vi "ERR Error Handler.vi"(0 "Error Status":bool, 5 "Error Code":i32, 7 "Cause Of Error":string, 9 "Error Source In":string="SubVI", 11 "Error In (no error)":errorcluster, 12 "Previous Error In (no Error)":errorcluster={"status"=FALSE, "code"=0, "source"="Empty"}) -> (15 "Error Out":errorcluster)   [LabVIEW 2012]
doc: "This VI has two modes: Error Handler Mode, and User Error Mode.\nWhen the error flag is FALSE then the vi functions as an error has not ocurred then the error cluster is passed through. If an error has ocurred then it will handle the error. If a previous error has not ocurred and the Error Flag is TRUE then the VI will assert the error and pass it through.\n\nUpon asserting a user error the vi checks to see if the New Error Code corresponds to one in the initialized error code array if it does not find it then it will use error code 9999 and state the \"Error Not In Error File\" message within the source text. This may be because of an incorrect error code, an error code not entered in the ErrorDescription.ini file or an unitialized error operation.\n\nThe error source will contain the date, time, error description, cause of error (if entered), and the call chain of the error occurrence.\n\nIf an error is flagged that is not present in the error description file (e.g., it is a labview error) then an automatic dialog box is opened. If a user error is found then a dialog box will be opened only if the error level is not '0'. If the error level is greater than 1 then the error handling is bypassed (i.e., the error is not recovered and is passed though).\n\nThe error will be logged always or the first time it is handled in pass through mode (level=0).\n\nIf the erro level is '2' then a 3 button dialog will be called in order for the user to select: Recover, Pass Through, or Stop. The VI will log the users selection as well as any additional comments in the recovery line of the error log. It will then take the appropriate action depending on the dialog choice.\n\nThis vi was created by David Gianetto, contact me with any problems, questions, etc."
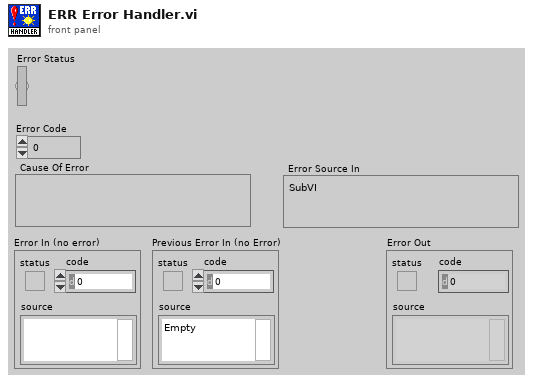
[diagram p1: front panel]
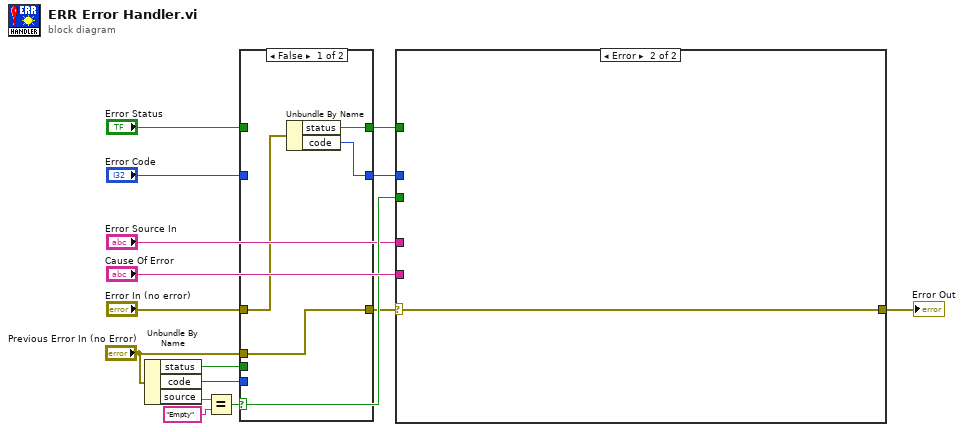
[diagram p0: block diagram]
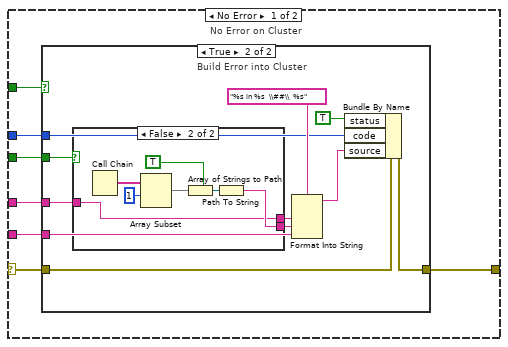
[diagram p3: hidden frame]
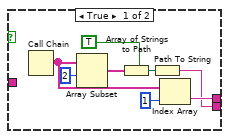
[diagram p5: hidden frame]
diagram:
  n1 = Unbundle By Name("Previous Error In (no Error)") -> ("status"=w7:bool, "code"=w6:i32, "source"=w13:string)
  n2 = Equal?(x=w13, y="Empty") -> (x = y?=w5:bool)
  n3 = case shown="False" w5 {
    tunnel: [w16 w22] -> w3
    tunnel: "Error Status" -> [_ w22]
    tunnel: [w17 w21] -> w2
    tunnel: "Error Code" -> [_ w21]
    tunnel: [w19 w20] -> w1
    tunnel: "Error In (no error)" -> [w18 w20]
    tunnel: w7 -> [_ _]
    tunnel: w6 -> [_ _]
    tunnel: "Previous Error In (no Error)" -> [w19 _]
    frame False {
      n4 = Unbundle By Name(w18) -> ("status"=w16:bool, "code"=w17:i32)
    }
    frame True {
    }
  }
  n5 = case shown="Error" w1 {
    selector: w1 -> [w23 w57]
    tunnel: [w27 w57] -> w15
    tunnel: w3 -> [w26 _]
    tunnel: w2 -> [w29 _]
    tunnel: "Cause Of Error" -> [w28 _]
    tunnel: w5 -> [w25 _]
    tunnel: "Error Source In" -> [w24 _]
    frame No Error {
      # "No Error on Cluster"
      n6 = case shown="True" w26 {
        tunnel: w29 -> [_ w34]
        tunnel: w28 -> [_ w33]
        tunnel: [errorcluster {"status"=FALSE, "code"=0, "source"=""} ("Error In (no error)") w40] -> w27
        tunnel: w23 -> [_ w39]
        tunnel: w25 -> [_ w32]
        tunnel: w24 -> [_ w31]
        frame False {
          # "No Error"
        }
        frame True {
          # "Build Error into Cluster"
          n7 = case shown="False" w32 {
            tunnel: [w43 w50] -> w38
            tunnel: [w42 w52] -> w35
            tunnel: w31 -> [_ w50]
            frame True {
              n8 = Call Chain() -> (call chain=w45:string[])
              n9 = Array Subset(array=w45, index=2) -> (w47:string[])  [unwired: 1 in]
              n10 = Array of Strings to Path(0:w47, 1:TRUE ("relative")) -> (2:w49:path)
              n11 = Path To String(path=w49) -> (string=w42:string)
              n12 = Index Array(array=w45, index=1) -> (element=w43:string)
            }
            frame False {
              n13 = Call Chain() -> (call chain=w51:string[])
              n14 = Array Subset(array=w51, index=1) -> (w54:string[])  [unwired: 1 in]
              n15 = Array of Strings to Path(0:w54, 1:TRUE ("relative")) -> (2:w56:path)
              n16 = Path To String(path=w56) -> (string=w52:string)
            }
          }
          n17 = Format Into String(format string="%s in %s  \\##\\  %s", w38, w35, w33) -> (resulting string=w36:string)  [unwired: 2 in, 1 out]
          n18 = Bundle By Name(cluster=w39, "status"=TRUE, "code"=w34, "source"=w36) -> (w40:errorcluster)
        }
      }
    }
    frame Error {
    }
  }
  "Error Out" <- w15
